vi "AdjustO3_170926.vi"(0 "CONTROL METHOD":bool, 1 "O3 Generator Control":T1={"Gen Output 0, Imin (mA)"=4.0, "USB3102 Number"=0.0, "DO O3 Gen Power"=0, "AO O3 Gen"=0, "O3 Gen Limit, Imax (mA)"=20.0, "Smoothing factor 0<1"=0.2} {"Smoothing factor 0<1" min=0.0 max=1.0 step=0.01; "AO O3 Gen" min=0 max=2 step=1; "DO O3 Gen Power" min=0 max=7 step=1}, 4 "Control \nO3":dbl=20.0, 5 "Target (ppb)":i32=200, 7 "Control in":dbl, 9 "Ambient\nO3":dbl format="%0.2f", 11 "O3 ON":bool=TRUE) -> (10 "Plot O3 Generator Control %":dbl(slide) min=0.0 max=100.0 scale=0.0..100.0, 15 "Control out":dbl)   [LabVIEW 2017]
panel:
  # "O3 GENERATOR \nCONTROL SETTINGS"
  # "USB 3102 Channel Numbers"
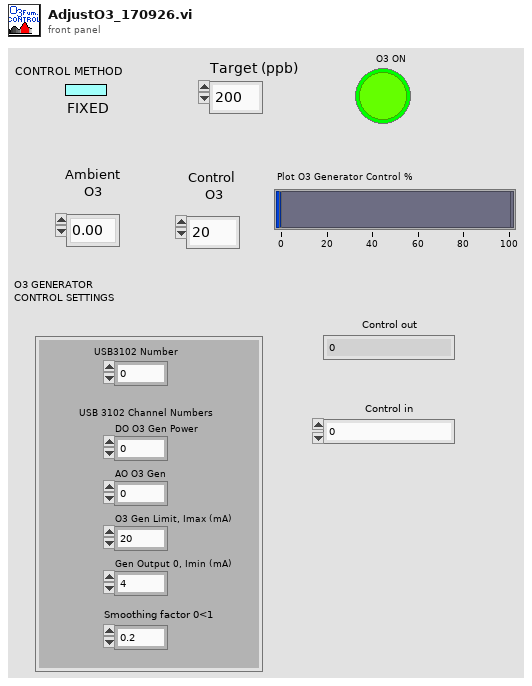
[diagram p1: front panel]
types:
  T1 = cluster{"Gen Output 0, Imin (mA)":sgl, "USB3102 Number":dbl, "DO O3 Gen Power":i32, "AO O3 Gen":i16, "O3 Gen Limit, Imax (mA)":dbl, "Smoothing factor 0<1":dbl}
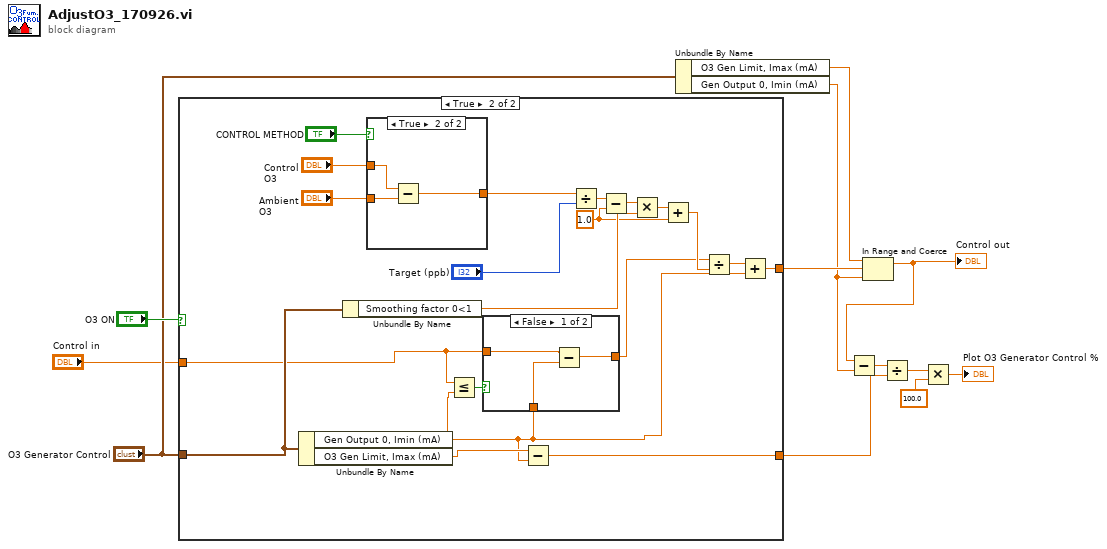
[diagram p0: block diagram]
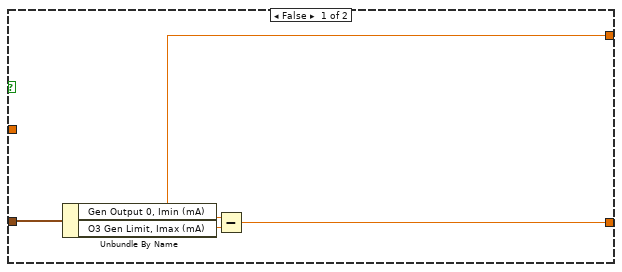
[diagram p2: hidden frame]
diagram:
  n1 = case shown="True" "O3 ON" {
    tunnel: "O3 Generator Control" -> [w15 w31]
    tunnel: [w14 w28] -> w9
    tunnel: [w13 w27] -> w6
    tunnel: "Control in" -> [_ w17]
    frame False {
      n2 = Unbundle By Name(w15) -> ("Gen Output 0, Imin (mA)"=w14:sgl, "O3 Gen Limit, Imax (mA)"=w16:dbl)
      n3 = Subtract(x=w16, y=w14) -> (x-y=w13:dbl)
    }
    frame True {
      w23 = 1.0 ("y")
      n4 = Unbundle By Name(w31) -> ("Gen Output 0, Imin (mA)"=w18:sgl, "O3 Gen Limit, Imax (mA)"=w30:dbl)
      n5 = Unbundle By Name(w31) -> ("Smoothing factor 0<1"=w32:dbl)
      n6 = case shown="True" "CONTROL METHOD" {
        tunnel: "Control \nO3" -> [w41 w44]
        tunnel: "Ambient\nO3" -> [_ w43]
        tunnel: [w41 w42] -> w29
        frame False {
        }
        frame True {
          n7 = Subtract(x=w44, y=w43) -> (x-y=w42:dbl)
        }
      }
      n8 = Less Or Equal?(x=w17, y=w18) -> (x <= y?=w19:bool)
      n9 = case shown="False" w19 {
        tunnel: w17 -> [w39 w40]
        tunnel: [w38 w40] -> w20
        tunnel: w18 -> [w37 _]
        frame False {
          n10 = Subtract(x=w39, y=w37) -> (x-y=w38:dbl)
        }
        frame True {
        }
      }
      n11 = Subtract(x=w30, y=w18) -> (x-y=w27:dbl)
      n12 = Divide(x=w29, y="Target (ppb)") -> (x/y=w26:dbl)
      n13 = Subtract(x=w26, y=w23) -> (x-y=w25:dbl)
      n14 = Multiply(x=w25, y=w32) -> (x*y=w24:dbl)
      n15 = Add(x=w24, y=w23) -> (x+y=w22:dbl)
      n16 = Divide(x=w20, y=w22) -> (x/y=w21:dbl)
      n17 = Add(x=w21, y=w18) -> (x+y=w28:dbl)
    }
  }
  n18 = Unbundle By Name("O3 Generator Control") -> ("O3 Gen Limit, Imax (mA)"=w10:dbl, "Gen Output 0, Imin (mA)"=w8:sgl)
  n19 = In Range and Coerce(upper limit=w10, x=w9, lower limit=w8) -> (coerced(x)=w1:dbl)  [unwired: 1 out]
  "Control out" <- w1
  n20 = Subtract(x=w1, y=w8) -> (x-y=w7:dbl)
  n21 = Divide(x=w7, y=w6) -> (x/y=w5:dbl)
  n22 = Multiply(x=w5, y=100.0) -> (x*y=→"Plot O3 Generator Control %":dbl)
